vi "Add.vi"(7 "top tree? (true)":bool=TRUE, 8 "error in (no error)":errorcluster, 10 "ProjectItem Refnum":refnum<vi>, 11 "SDIST in":refnum<class "NI_AB_API_SDIST.lvclass">) -> (0 "error out":errorcluster, 3 "SDIST out":refnum<class "NI_AB_API_SDIST.lvclass">)   [LabVIEW 2020, in "NI_AB_API_SDIST.lvclass"]
uses:
  <vilib>/AppBuilder/AB_API/SDIST/NI_AB_API_SDIST.lvclass
  <vilib>/AppBuilder/AB_API/SDIST/NI_AB_API_SDIST.lvclass/NI_AB_API_SDIST.ctl
  <vilib>/AppBuilder/AB_Classes/Source/AB_Source.lvclass
  <vilib>/AppBuilder/AB_Classes/Build/AB_Build.lvclass
  <vilib>/AppBuilder/AB_API/Build/NI_AB_API_Build.lvclass
  <vilib>/AppBuilder/AB_Classes/SourceDistribution/AB_SourceDistribution.lvclass
  e:/builds/penguin/labview/branches/2020/dev/dist/vi.lib/AppBuilder/AB_API/Build/NI_AB_API_Build.lvclass
  e:/builds/penguin/labview/branches/2020/dev/dist/vi.lib/AppBuilder/AB_API/SDIST/NI_AB_API_SDIST.lvclass
  e:/builds/penguin/labview/branches/2020/dev/dist/vi.lib/AppBuilder/AB_Classes/Build/AB_Build.lvclass
  e:/builds/penguin/labview/branches/2020/dev/dist/vi.lib/AppBuilder/AB_Classes/SourceDistribution/AB_SourceDistribution.lvclass
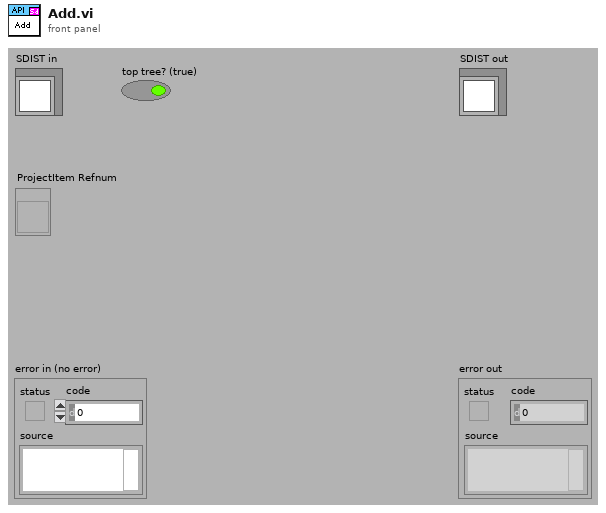
[diagram p1: front panel]
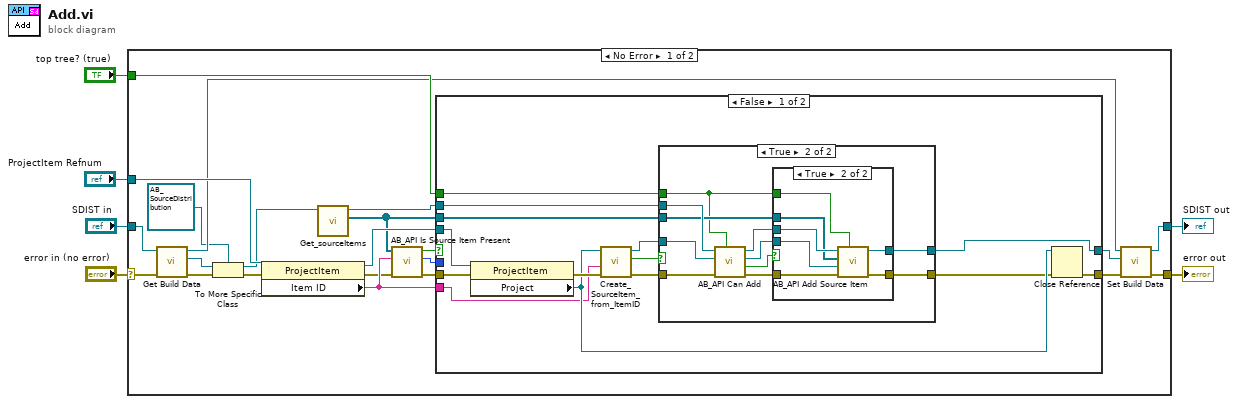
[diagram p0: block diagram]
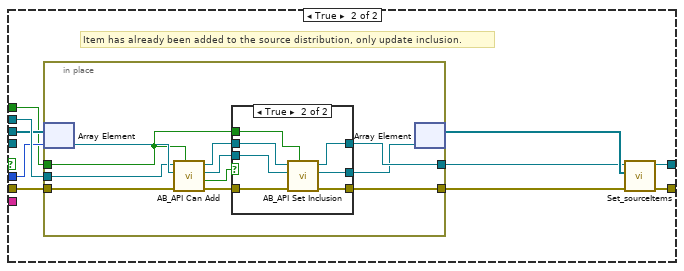
[diagram p4: hidden frame]
diagram:
  n1 = case shown="No Error" "error in (no error)" {
    selector: "error in (no error)" -> [w17 w97]
    tunnel: [w12 w97] -> w5
    tunnel: [w13 w96] -> w3
    tunnel: "SDIST in" -> [w18 w96]
    tunnel: "ProjectItem Refnum" -> [w28 _]
    tunnel: "top tree? (true)" -> [w27 _]
    frame No Error {
      n2 = call <vilib>:"Get Build Data.vi"("error in (no error)"=w17, "NI_AB_API_Build in"=w18) -> ("error out"=w8:errorcluster, "AB_Build.lvclass"=w16:refnum<class "AB_Build.lvclass">, "NI_AB_API_Build out"=w14:refnum<class "NI_AB_API_SDIST.lvclass">)  [unwired: 7 in]
      n3 = To More Specific Class(target class=refnum<class "AB_SourceDistribution.lvclass"> refnum ("AB_SourceDistribution.lvclass"), reference=w16, error in=w8) -> (specific class reference=w9:refnum<class "AB_SourceDistribution.lvclass">, error out=w7:errorcluster)
      n4 = property class="ProjectItem"(reference=w28, error in=w7) -> (reference out=w26:refnum<vi>, error out=w23:errorcluster, "Item ID"=w25:string)
      n5 = call <vilib>:"Get_sourceItems.vi"("Class in"=w9) -> ("sourceItems"=w21:refnum<class "AB_Source.lvclass">[], "Class out"=w22:refnum<class "AB_SourceDistribution.lvclass">)  [unwired: 8 in, 1 out]
      n6 = call <vilib>:"AB_API Is Source Item Present.vi"("error in"=w23, "item ID"=w25, "source items"=w21) -> ("error out"=w24:errorcluster, "index"=w19:i32, "source item present?"=w20:bool)  [unwired: 6 in]
      n7 = case shown="False" w20 {
        tunnel: w26 -> [w42 _]
        tunnel: [w38 w68] -> w15
        tunnel: [w34 w66] -> w11
        tunnel: w24 -> [w33 w72]
        tunnel: w22 -> [w32 w74]
        tunnel: w25 -> [w31 _]
        tunnel: w21 -> [w30 w73]
        tunnel: w19 -> [_ w71]
        tunnel: w27 -> [w29 w65]
        frame False {
          n8 = property class="ProjectItem"(reference=w42, error in=w33) -> (error out=w41:errorcluster, "Project"=w36:refnum<vi>)  [unwired: 1 out]
          n9 = call <vilib>:"Create_SourceItem_from_ItemID.vi"("error in (no error)"=w41, "itemID"=w31, "Project Refnum"=w36) -> ("error out"=w39:errorcluster, "valid?"=w37:bool, "AB_Source out"=w40:refnum<class "AB_Source.lvclass">)  [unwired: 6 in]
          n10 = case shown="True" w37 {
            tunnel: w40 -> [_ w49]
            tunnel: w39 -> [w43 w50]
            tunnel: w32 -> [w44 w55]
            tunnel: [w44 w54] -> w38
            tunnel: [w43 w53] -> w35
            tunnel: w30 -> [_ w52]
            tunnel: w29 -> [_ w51]
            frame False {
            }
            frame True {
              n11 = call <vilib>:"AB_API Can Add.vi"("top tree? (true)"=w51, "error in (no error)"=w50, "AB_Source in"=w49, "Build in"=w55) -> ("error out"=w46:errorcluster, "can add?"=w45:bool, "AB_Source out"=w48:refnum<class "AB_Source.lvclass">, "Build out"=w47:refnum<class "AB_SourceDistribution.lvclass">)  [unwired: 4 in]
              n12 = case shown="True" w45 {
                tunnel: [w57 w64] -> w53
                tunnel: w46 -> [w57 w63]
                tunnel: [w56 w62] -> w54
                tunnel: w47 -> [w56 w61]
                tunnel: w48 -> [_ w60]
                tunnel: w52 -> [_ w59]
                tunnel: w51 -> [_ w58]
                frame False {
                }
                frame True {
                  n13 = call <vilib>:"AB_API Add Source Item.vi"("top tree? (true)"=w58, "error in"=w63, "Source in"=w60, "source items"=w59, "Build in"=w61) -> ("error out"=w64:errorcluster, "Build out"=w62:refnum<class "AB_SourceDistribution.lvclass">)  [unwired: 5 in]
                }
              }
            }
          }
          n14 = Close Reference(reference=w36, error in (no error)=w35) -> (error out=w34:errorcluster)
        }
        frame True {
          # "Item has already been added to the source distribution, only update inclusion."
          n15 = in-place {
            in-place-border: [w85] -> w69
            in-place-border: w74 -> [w80]
            in-place-border: w72 -> [w78]
            in-place-border: [w84] -> w67
            in-place-border: w65 -> [w75]
            n16 = in-place-array #1(w73, w71) -> (w82:refnum<class "AB_Source.lvclass">)
            n17 = call <vilib>:"AB_API Can Add.vi"("top tree? (true)"=w75, "error in (no error)"=w78, "AB_Source in"=w82, "Build in"=w80) -> ("error out"=w77:errorcluster, "can add?"=w76:bool, "AB_Source out"=w81:refnum<class "AB_Source.lvclass">, "Build out"=w79:refnum<class "AB_SourceDistribution.lvclass">)  [unwired: 4 in]
            n18 = case shown="True" w76 {
              tunnel: [w86 w90] -> w84
              tunnel: [w88 w95] -> w85
              tunnel: w79 -> [w88 w93]
              tunnel: w81 -> [w87 w92]
              tunnel: w77 -> [w86 w91]
              tunnel: [w87 w94] -> w83
              tunnel: w75 -> [_ w89]
              frame False {
              }
              frame True {
                n19 = call <vilib>:"AB_API Set Inclusion.vi"("top tree? (true)"=w89, "error in (no error)"=w91, "Source in"=w92, "Build in"=w93) -> ("error out"=w90:errorcluster, "AB_Source_VI out"=w94:refnum<class "AB_Source.lvclass">, "AB_Build out"=w95:refnum<class "AB_SourceDistribution.lvclass">)  [unwired: 5 in]
              }
            }
            n20 = in-place-array #1(w83) -> (w70:refnum<class "AB_Source.lvclass">[])  [unwired: 1 out]
          }
          n21 = call <vilib>:"Set_sourceItems.vi"("error in (no error)"=w67, "sourceItems"=w70, "Class in"=w69) -> ("error out"=w66:errorcluster, "Class out"=w68:refnum<class "AB_SourceDistribution.lvclass">)  [unwired: 7 out]
        }
      }
      n22 = call <vilib>:"Set Build Data.vi"("error in (no error)"=w11, "AB_Build.lvclass"=w15, "NI_AB_API_Build in"=w14) -> ("error out"=w12:errorcluster, "NI_AB_API_Build out"=w13:refnum<class "NI_AB_API_SDIST.lvclass">)  [unwired: 7 in]
    }
    frame Error {
    }
  }
  "error out" <- w5
  "SDIST out" <- w3
